vi "write_coef_init.vi"(8 "error in (no error)":errorcluster, 10 "coef_init":dbl[][](array[numeric]), 11 "SGDRegressor in":refnum<class "SGDRegressor.lvclass">) -> (0 "error out":errorcluster, 3 "SGDRegressor out":refnum<class "SGDRegressor.lvclass">)   [LabVIEW 2020, in "SGDRegressor.lvclass"]
uses:
  SGDRegressor.lvclass
  SGDRegressor.lvclass/SGDRegressor.ctl
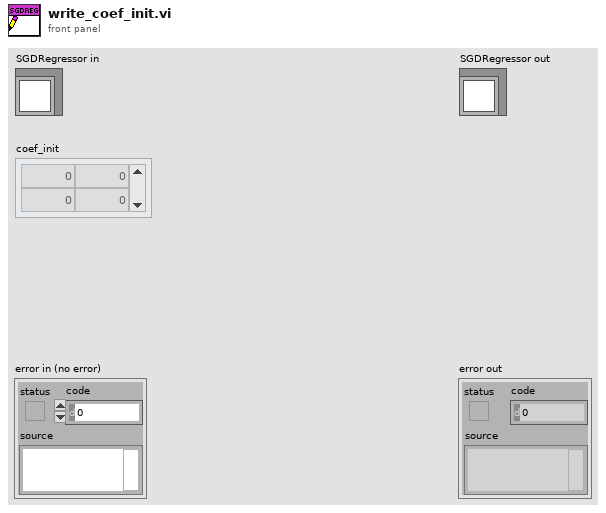
[diagram p1: front panel]
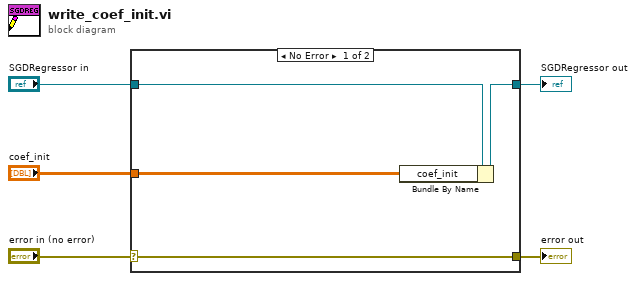
[diagram p0: block diagram]
diagram:
  n1 = case shown="No Error" "error in (no error)" {
    selector: "error in (no error)" -> [w9 w10]
    tunnel: [w9 w10] -> w4
    tunnel: [w7 w11] -> w2
    tunnel: "SGDRegressor in" -> [w8 w11]
    tunnel: "coef_init" -> [w6 _]
    frame No Error {
      n2 = Bundle By Name(cluster=w8, "coef_init"=w6) -> (w7:refnum<class "SGDRegressor.lvclass">)
    }
    frame Error {
    }
  }
  "error out" <- w4
  "SGDRegressor out" <- w2
